vi "逆向空载试验判定.vi"(7 "Result":refnum<vi>, 10 "判定参数":T1, 11 "XY曲线":cluster{"X":dbl[], "Y":dbl[]}[](array[cluster])) -> (2 "判定项长度":i32, 3 "OK？":bool)   [LabVIEW 2020]
uses:
  <userlib>/_MGI/1D Array/MGI Average/MGI Average (DBL[]).vi
panel:
  out "逆向平均值":dbl
  out "正向平均值":dbl
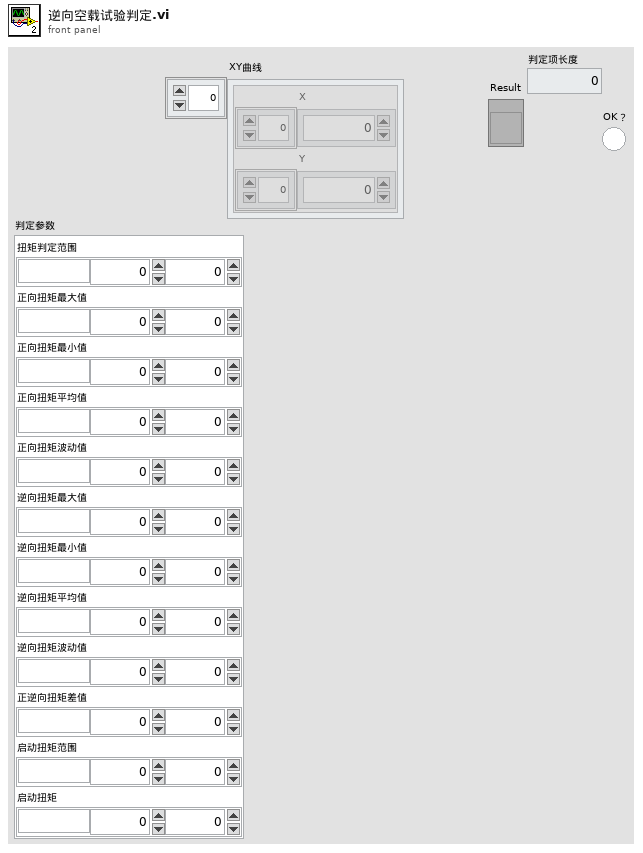
[diagram p1: front panel]
types:
  T1 = cluster{"扭矩判定范围":cluster{"单位":string, "下限":dbl, "上限":dbl}, "正向扭矩最大值":cluster{"单位":string, "下限":dbl, "上限":dbl}, "正向扭矩最小值":cluster{"单位":string, "下限":dbl, "上限":dbl}, "正向扭矩平均值":cluster{"单位":string, "下限":dbl, "上限":dbl}, "正向扭矩波动值":cluster{"单位":string, "下限":dbl, "上限":dbl}, "逆向扭矩最大值":cluster{"单位":string, "下限":dbl, "上限":dbl}, "逆向扭矩最小值":cluster{"单位":string, "下限":dbl, "上限":dbl}, "逆向扭矩平均值":cluster{"单位":string, "下限":dbl, "上限":dbl}, "逆向扭矩波动值":cluster{"单位":string, "下限":dbl, "上限":dbl}, "正逆向扭矩差值":cluster{"单位":string, "下限":dbl, "上限":dbl}, "启动扭矩范围":cluster{"单位":string, "下限":dbl, "上限":dbl}, "启动扭矩":cluster{"单位":string, "下限":dbl, "上限":dbl}}
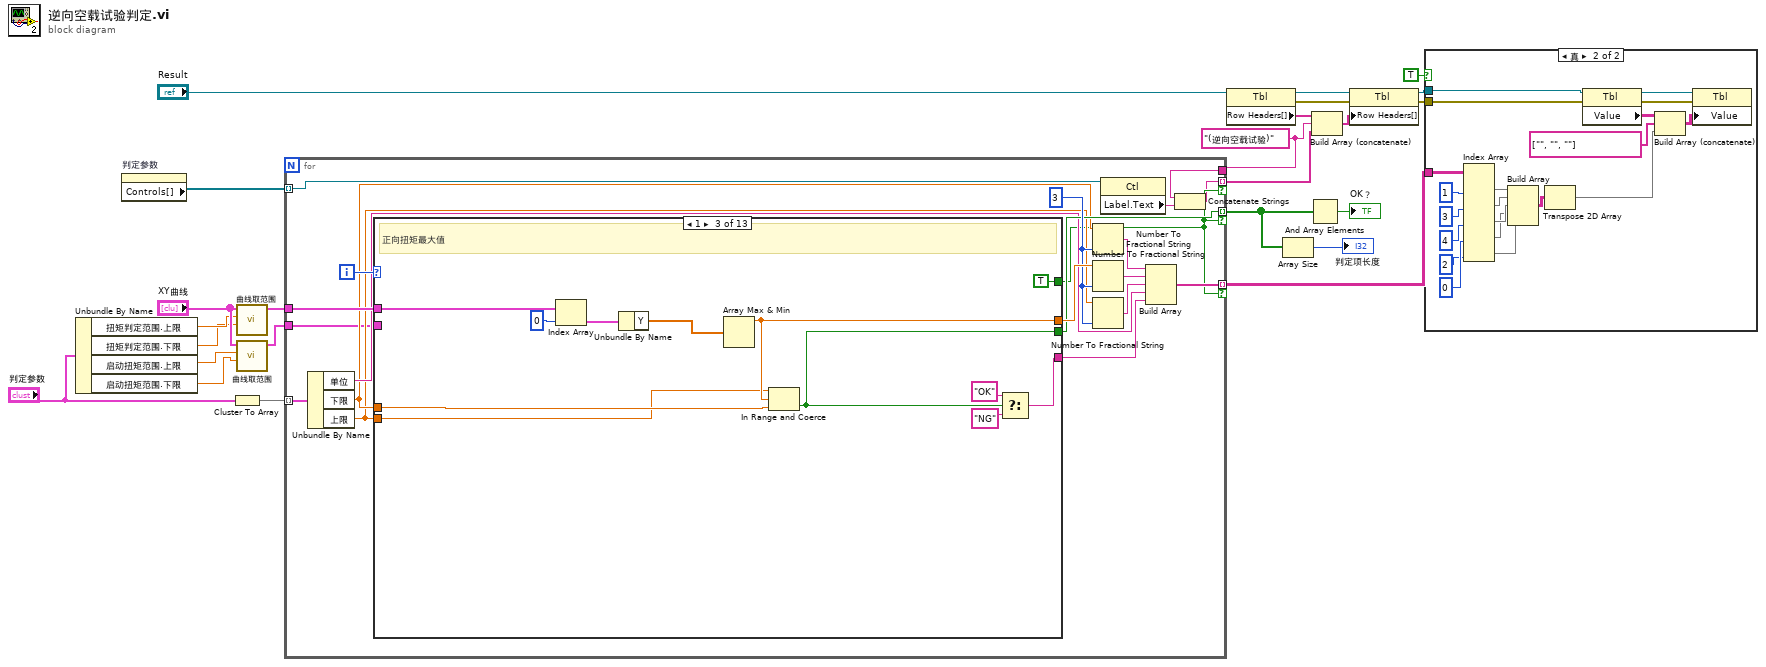
[diagram p0: block diagram]
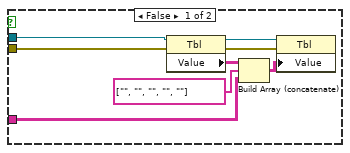
[diagram p2: hidden frame]
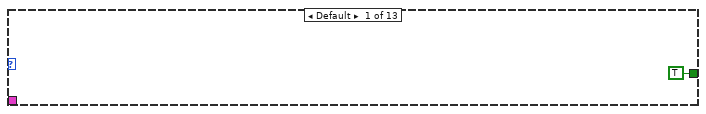
[diagram p3: hidden frame]
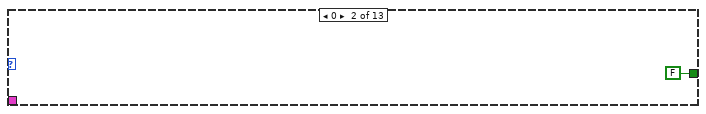
[diagram p4: hidden frame]
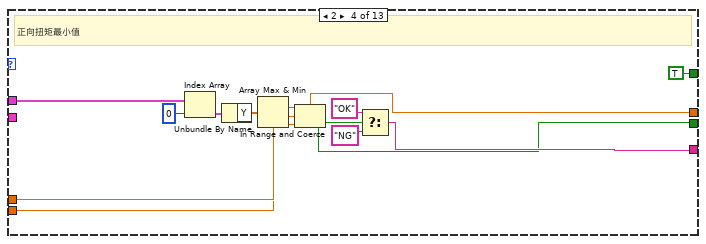
[diagram p5: hidden frame]
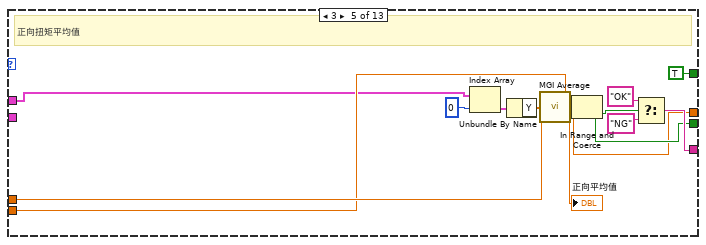
[diagram p6: hidden frame]
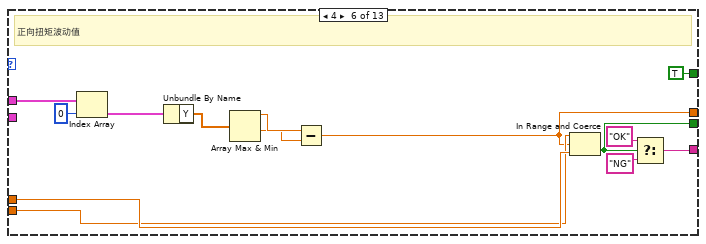
[diagram p7: hidden frame]
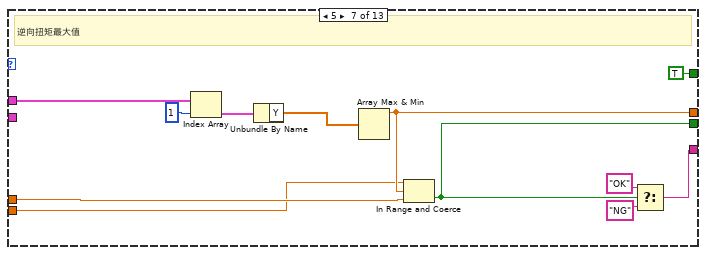
[diagram p8: hidden frame]
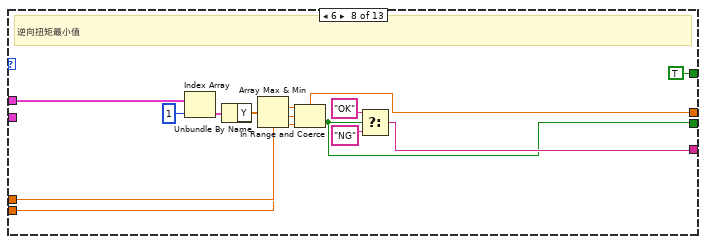
[diagram p9: hidden frame]
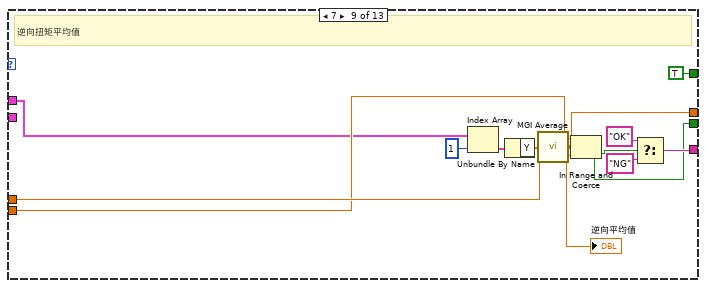
[diagram p10: hidden frame]
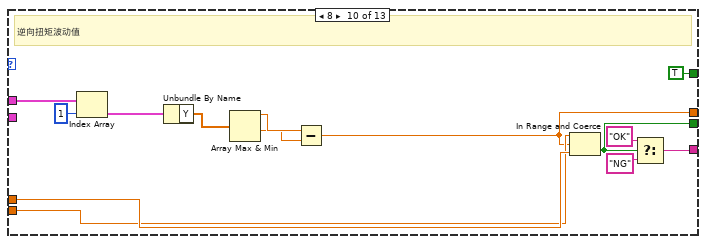
[diagram p11: hidden frame]
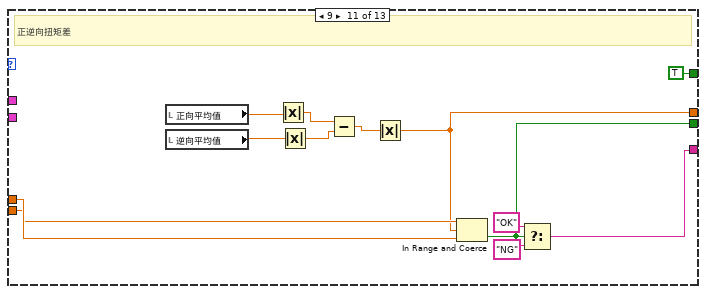
[diagram p12: hidden frame]
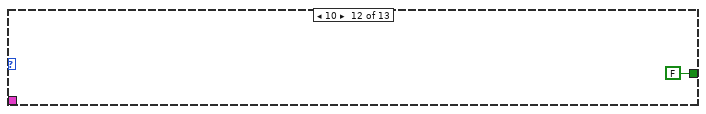
[diagram p13: hidden frame]
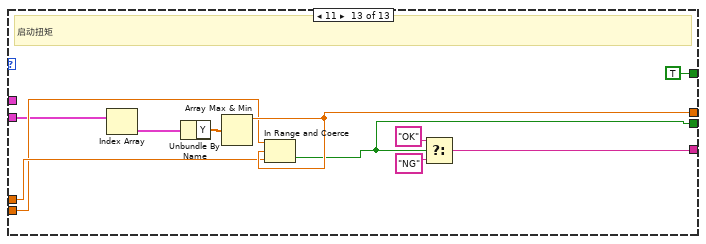
[diagram p14: hidden frame]
diagram:
  w10 = "(逆向空载试验)" ("Label.Text")
  n1 = Unbundle By Name("判定参数") -> ("扭矩判定范围.上限"=w4:dbl, "扭矩判定范围.下限"=w3:dbl, "启动扭矩范围.上限"=w2:dbl, "启动扭矩范围.下限"=w1:dbl)
  n2 = property on="判定参数" class="Clust (严格)"() -> ("Controls[]"=w6:refnum<vi>[])  [unwired: 2 in, 2 out]
  n3 = Cluster To Array(cluster="判定参数") -> (array=w24:cluster{"单位":string, "下限":dbl, "上限":dbl}[])
  n4 = call "曲线取范围.vi"("下限"=w3, "上限"=w4, "曲线In"="XY曲线") -> ("曲线Out"=w9:cluster{"X":dbl[], "Y":dbl[]}[])  [unwired: 8 in]
  n5 = call "曲线取范围.vi"("下限"=w1, "上限"=w2, "曲线In"="XY曲线") -> ("曲线Out"=w8:cluster{"X":dbl[], "Y":dbl[]}[])  [unwired: 8 in]
  n6 = for {
    tunnel: w24 -> [w44] mode=indexing
    tunnel: w6 -> [w42] mode=indexing
    tunnel: w9 -> [w40]
    tunnel: [w34] -> w12 mode=indexing if=w28
    tunnel: [w30] -> w14 mode=indexing if=w28
    tunnel: [w27] -> w17 mode=indexing if=w28
    tunnel: w10 -> [w26]
    tunnel: w8 -> [w25]
    i -> [w43]
    w39 = i16 3 ("精度(6)")
    n7 = Unbundle By Name(w44) -> ("单位"=w33:string, "下限"=w32:dbl, "上限"=w31:dbl)
    n8 = case shown="1" w43 {
      tunnel: [_ _ w55 w61 w71 w83 w105 w111 w121 w133 w147 _ w167] -> w41
      tunnel: w40 -> [_ _ w58 w70 w75 w89 w108 w120 w125 w139 _ _ _]
      tunnel: [_ _ w52 w66 w80 w94 w102 w116 w130 w144 w149 _ w166] -> w35
      tunnel: [_ _ w51 w65 w79 w93 w101 w115 w129 w143 w148 _ w165] -> w34
      tunnel: w32 -> [_ _ w50 w64 w78 w92 w100 w114 w128 w142 w156 _ w163]
      tunnel: w31 -> [_ _ w49 w63 w77 w91 w99 w113 w127 w141 w155 _ w162]
      tunnel: [TRUE FALSE TRUE TRUE TRUE TRUE TRUE TRUE TRUE TRUE TRUE FALSE TRUE] -> w28
      tunnel: w25 -> [_ _ _ _ _ _ _ _ _ _ _ _ w161]
      frame Default {
      }
      frame 0 {
      }
      frame 1 {
        # "正向扭矩最大值"
        n9 = Index Array(array=w58, index=0 ("索引")) -> (element=w56:cluster{"X":dbl[], "Y":dbl[]})
        n10 = Unbundle By Name(w56) -> ("Y"=w47:dbl[])
        n11 = Array Max & Min(array=w47) -> (max value=w55:dbl)  [unwired: 3 out]
        n12 = In Range and Coerce(upper limit=w49, x=w55, lower limit=w50) -> (In Range?=w51:bool)  [unwired: 1 out]
        n13 = Select(t="OK", s=w51, f="NG") -> (s? t:f=w52:string)
      }
      frame 2 {
        # "正向扭矩最小值"
        n14 = Index Array(array=w70, index=0 ("索引")) -> (element=w69:cluster{"X":dbl[], "Y":dbl[]})
        n15 = Unbundle By Name(w69) -> ("Y"=w60:dbl[])
        n16 = Array Max & Min(array=w60) -> (min value=w61:dbl)  [unwired: 3 out]
        n17 = In Range and Coerce(upper limit=w63, x=w61, lower limit=w64) -> (In Range?=w65:bool)  [unwired: 1 out]
        n18 = Select(t="OK", s=w65, f="NG") -> (s? t:f=w66:string)
      }
      frame 3 {
        # "正向扭矩平均值"
        n19 = Index Array(array=w75, index=0 ("索引")) -> (element=w74:cluster{"X":dbl[], "Y":dbl[]})
        n20 = Unbundle By Name(w74) -> ("Y"=w73:dbl[])
        n21 = call-poly <userlib>:"MGI Average.vi"("Double[]"=w73) -> ("Average"=w71:dbl)  [unwired: 1 in]
        "正向平均值" <- w71
        n22 = In Range and Coerce(upper limit=w77, x=w71, lower limit=w78) -> (In Range?=w79:bool)  [unwired: 1 out]
        n23 = Select(t="OK", s=w79, f="NG") -> (s? t:f=w80:string)
      }
      frame 4 {
        # "正向扭矩波动值"
        n24 = Index Array(array=w89, index=0 ("索引")) -> (element=w88:cluster{"X":dbl[], "Y":dbl[]})
        n25 = Unbundle By Name(w88) -> ("Y"=w86:dbl[])
        n26 = Array Max & Min(array=w86) -> (max value=w85:dbl, min value=w84:dbl)  [unwired: 2 out]
        n27 = Subtract(x=w85, y=w84) -> (x-y=w83:dbl)
        n28 = In Range and Coerce(upper limit=w91, x=w83, lower limit=w92) -> (In Range?=w93:bool)  [unwired: 1 out]
        n29 = Select(t="OK", s=w93, f="NG") -> (s? t:f=w94:string)
      }
      frame 5 {
        # "逆向扭矩最大值"
        n30 = Index Array(array=w108, index=1 ("索引")) -> (element=w106:cluster{"X":dbl[], "Y":dbl[]})
        n31 = Unbundle By Name(w106) -> ("Y"=w97:dbl[])
        n32 = Array Max & Min(array=w97) -> (max value=w105:dbl)  [unwired: 3 out]
        n33 = In Range and Coerce(upper limit=w99, x=w105, lower limit=w100) -> (In Range?=w101:bool)  [unwired: 1 out]
        n34 = Select(t="OK", s=w101, f="NG") -> (s? t:f=w102:string)
      }
      frame 6 {
        # "逆向扭矩最小值"
        n35 = Index Array(array=w120, index=1 ("索引")) -> (element=w119:cluster{"X":dbl[], "Y":dbl[]})
        n36 = Unbundle By Name(w119) -> ("Y"=w110:dbl[])
        n37 = Array Max & Min(array=w110) -> (min value=w111:dbl)  [unwired: 3 out]
        n38 = In Range and Coerce(upper limit=w113, x=w111, lower limit=w114) -> (In Range?=w115:bool)  [unwired: 1 out]
        n39 = Select(t="OK", s=w115, f="NG") -> (s? t:f=w116:string)
      }
      frame 7 {
        # "逆向扭矩平均值"
        n40 = Index Array(array=w125, index=1 ("索引")) -> (element=w124:cluster{"X":dbl[], "Y":dbl[]})
        n41 = Unbundle By Name(w124) -> ("Y"=w123:dbl[])
        n42 = call-poly <userlib>:"MGI Average.vi"("Double[]"=w123) -> ("Average"=w121:dbl)  [unwired: 1 in]
        "逆向平均值" <- w121
        n43 = In Range and Coerce(upper limit=w127, x=w121, lower limit=w128) -> (In Range?=w129:bool)  [unwired: 1 out]
        n44 = Select(t="OK", s=w129, f="NG") -> (s? t:f=w130:string)
      }
      frame 8 {
        # "逆向扭矩波动值"
        n45 = Index Array(array=w139, index=1 ("索引")) -> (element=w138:cluster{"X":dbl[], "Y":dbl[]})
        n46 = Unbundle By Name(w138) -> ("Y"=w136:dbl[])
        n47 = Array Max & Min(array=w136) -> (max value=w135:dbl, min value=w134:dbl)  [unwired: 2 out]
        n48 = Subtract(x=w135, y=w134) -> (x-y=w133:dbl)
        n49 = In Range and Coerce(upper limit=w141, x=w133, lower limit=w142) -> (In Range?=w143:bool)  [unwired: 1 out]
        n50 = Select(t="OK", s=w143, f="NG") -> (s? t:f=w144:string)
      }
      frame 9 {
        # "正逆向扭矩差"
        n51 = local read "正向平均值"() -> (w154:dbl)
        n52 = local read "逆向平均值"() -> (w153:dbl)
        n53 = Absolute Value(x=w154) -> (abs(x)=w152:dbl)
        n54 = Absolute Value(x=w153) -> (abs(x)=w151:dbl)
        n55 = Subtract(x=w152, y=w151) -> (x-y=w150:dbl)
        n56 = Absolute Value(x=w150) -> (abs(x)=w147:dbl)
        n57 = In Range and Coerce(upper limit=w155, x=w147, lower limit=w156) -> (In Range?=w148:bool)  [unwired: 1 out]
        n58 = Select(t="OK", s=w148, f="NG") -> (s? t:f=w149:string)
      }
      frame 10 {
      }
      frame 11 {
        # "启动扭矩"
        n59 = Index Array(array=w161) -> (element=w171:cluster{"X":dbl[], "Y":dbl[]})  [unwired: 1 in]
        n60 = Unbundle By Name(w171) -> ("Y"=w170:dbl[])
        n61 = Array Max & Min(array=w170) -> (max value=w167:dbl)  [unwired: 3 out]
        n62 = In Range and Coerce(upper limit=w162, x=w167, lower limit=w163) -> (In Range?=w165:bool)  [unwired: 1 out]
        n63 = Select(t="OK", s=w165, f="NG") -> (s? t:f=w166:string)
      }
    }
    n64 = Number To Fractional String(number=w32, precision (6)=w39) -> (F-format string=w38:string)  [unwired: 2 in]
    n65 = Number To Fractional String(number=w41, precision (6)=w39) -> (F-format string=w37:string)  [unwired: 2 in]
    n66 = Number To Fractional String(number=w31, precision (6)=w39) -> (F-format string=w36:string)  [unwired: 2 in]
    n67 = property class="Ctl"(reference=w42) -> ("Label.Text"=w29:string)  [unwired: 1 in, 2 out]
    n68 = Build Array(w38, w37, w36, w33, w35) -> (w30:string[])
    n69 = Concatenate Strings(w26, w29) -> (w27:string)
  }
  n70 = property class="Tbl"(reference="Result") -> (reference out=w19:refnum<vi>, error out=w22:errorcluster, "Row Headers[]"=w15:string[])  [unwired: 1 in]
  n71 = Array Size(array=w12) -> (size(s)=→"判定项长度":i32)
  n72 = And Array Elements(Boolean array=w12) -> (logical AND=→"OK？":bool)
  n73 = Build Array (concatenate)(w15, w10, w17) -> (w18:string[])
  n74 = property class="Tbl"(reference=w19, error in=w22, "Row Headers[]"=w18) -> (reference out=w20:refnum<vi>, error out=w21:errorcluster)
  n75 = case shown="真" TRUE {
    tunnel: w21 -> [w177 w197]
    tunnel: w20 -> [w174 w194]
    tunnel: w14 -> [w173 w185]
    frame False {
      n76 = property class="Tbl"(reference=w174, error in=w177) -> (reference out=w175:refnum<vi>, error out=w176:errorcluster, "Value"=w178:string[][])
      n77 = Build Array (concatenate)(w178, string[] ["", "", "", "", ""], w173) -> (w179:string[][])
      n78 = property class="Tbl"(reference=w175, error in=w176, "Value"=w179) -> ()  [unwired: 2 out]
    }
    frame True {
      n79 = Index Array(array=w185, index (col) #1=1 ("禁用的索引 (列)"), index (col) #2=3 ("索引 (列)"), index (col) #3=4 ("索引 (列)"), index (col) #4=0 ("索引 (列)"), index (col) #5=2 ("索引 (列)")) -> (element #1=w189:string[], element #2=w188:string[], element #3=w187:string[], element #4=w181:string[], element #5=w180:string[])  [unwired: 5 in]
      n80 = Build Array(w189, w188, w187, w181, w180) -> (w186:string[][])
      n81 = Transpose 2D Array(2D array=w186) -> (transposed array=w184:string[][])
      n82 = property class="Tbl"(reference=w194, error in=w197) -> (reference out=w195:refnum<vi>, error out=w196:errorcluster, "Value"=w198:string[][])
      n83 = Build Array (concatenate)(w198, string[] ["", "", ""], w184) -> (w199:string[][])
      n84 = property class="Tbl"(reference=w195, error in=w196, "Value"=w199) -> ()  [unwired: 2 out]
    }
  }
